vi "DB_checkID_writeID_1.vi"() -> ()   [LabVIEW 2018]
uses:
  <vilib>/addons/database/Connection.llb/DB Tools Open Connec (Path).vi
  <vilib>/addons/database/NI_Database_API.lvlib
panel:
  out "error out":errorcluster
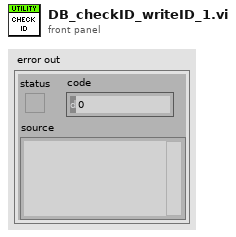
[diagram p1: front panel]
types:
  T1 = typedef "NI_Database_API.lvlib/Conn ObjectReference.ctl" = refnum<k1>
  T2 = typedef "Equipos_Medicion_cluster.ctl" = cluster{"ID_EQUIPO":i32, "IP_EQUIPO":string, "NOMBRE_EQUIPO":string, "ESTADO_EQUIPO":string, "DESCRIPCION":string, "ID_MEDICION":i32, "ESTADO_MEDICION":string, "TIEMPO_MEDICION":string}
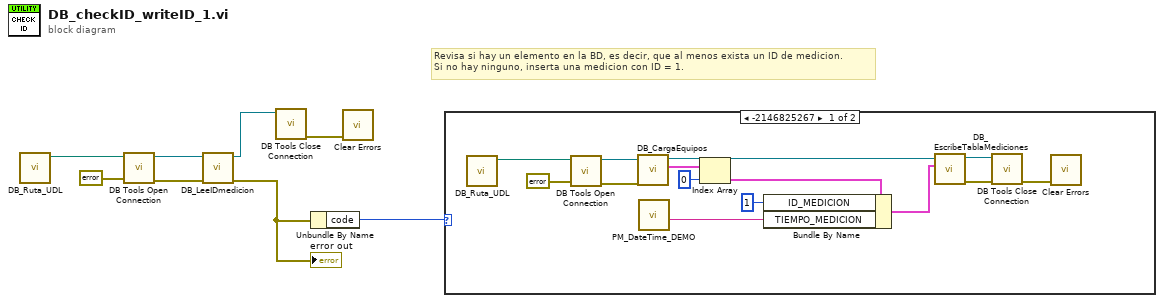
[diagram p0: block diagram]
diagram:
  # "Revisa si hay un elemento en la BD, es decir, que al menos exista un ID de medicion.\nSi no hay ninguno, inserta una medicion con ID = 1."
  n1 = call "DB_Ruta_UDL.vi"() -> ("UDL ruta"=w7:path)  [unwired: 11 in]
  n2 = call-poly <vilib>:"DB Tools Open Connection.vi"("error in (no error)"=errorcluster {"status"=FALSE, "code"=0, "source"=""}, "connection information"=w7) -> ("error out"=w5:errorcluster, "connection reference"=w6:T1)  [unwired: 6 in]
  n3 = call "DB_LeeIDmedicion.vi"("error in (no error)"=w5, "db in"=w6) -> ("error out"=w4:errorcluster, "db out"=w2:T1)  [unwired: 7 in, 1 out]
  "error out" <- w4
  n4 = call <vilib>:"DB Tools Close Connection.vi"("connection reference"=w2) -> ("error out"=w1:errorcluster)  [unwired: 6 in]
  n5 = Unbundle By Name(w4) -> ("code"=w3:i32)
  n6 = call <vilib>:"Clear Errors.vi"("error in (no error)"=w1) -> ()  [unwired: 5 in, 2 out]
  n7 = case shown="-2146825267" w3 {
    frame -2146825267 {
      n8 = call "DB_Ruta_UDL.vi"() -> ("UDL ruta"=w12:path)  [unwired: 11 in]
      n9 = call-poly <vilib>:"DB Tools Open Connection.vi"("error in (no error)"=errorcluster {"status"=FALSE, "code"=0, "source"=""}, "connection information"=w12) -> ("error out"=w9:errorcluster, "connection reference"=w10:T1)  [unwired: 6 in]
      n10 = call "DB_CargaEquipos.vi"("error in (no error)"=w9, "db in"=w10) -> ("Equipos_out"=w21:T2[], "db out"=w22:T1)  [unwired: 2 in, 6 out]
      n11 = call "PM_DateTime_DEMO.vi"() -> ("TIEMPO_MEDICION"=w13:string)  [unwired: 10 in, 1 out]
      n12 = Index Array(array=w21, index=0) -> (element=w20:T2)
      n13 = Bundle By Name(cluster=w20, "ID_MEDICION"=1 ("ID_EQUIPO"), "TIEMPO_MEDICION"=w13) -> (w18:T2)
      n14 = call "DB_EscribeTablaMediciones.vi"("Equipo_Medicion in"=w18, "db in"=w22) -> ("error out"=w17:errorcluster, "db out"=w16:T1)  [unwired: 8 in]
      n15 = call <vilib>:"DB Tools Close Connection.vi"("error in (no error)"=w17, "connection reference"=w16) -> ("error out"=w14:errorcluster)  [unwired: 5 in]
      n16 = call <vilib>:"Clear Errors.vi"("error in (no error)"=w14) -> ()  [unwired: 5 in, 2 out]
    }
    frame Default {
    }
  }
